vi "MCP23S17_Get.vi"(5 "RF":T1 items=["RF_0", "RF_1", "RF_2", "RF_3"], 6 "Addr":u32 format="%x", 7 "RFU":T2, 8 "Error_In":errorcluster, 10 "Auto_Sel_Rsrc?":bool=TRUE, 11 "VISA_Rsrc_In":refnum<visa-resource-name>) -> (0 "Error_Out":errorcluster, 2 "Data":u32 format="%x", 3 "VISA_Rsrc_Out":refnum<visa-resource-name>)   [LabVIEW 2018]
uses:
  Types/RFU.ctl
  Types/RF.ctl
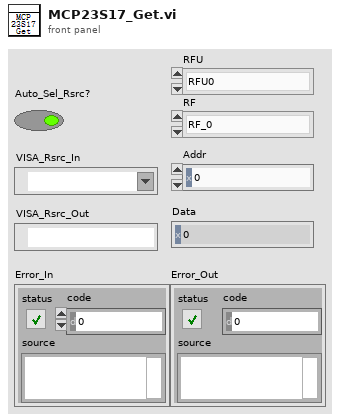
[diagram p1: front panel]
types:
  T1 = typedef "RF.ctl" = u16
  T2 = typedef "RFU.ctl" = enum8{"RFU0", "RFU1", "RFU2", "RFU3", "RFU4"}
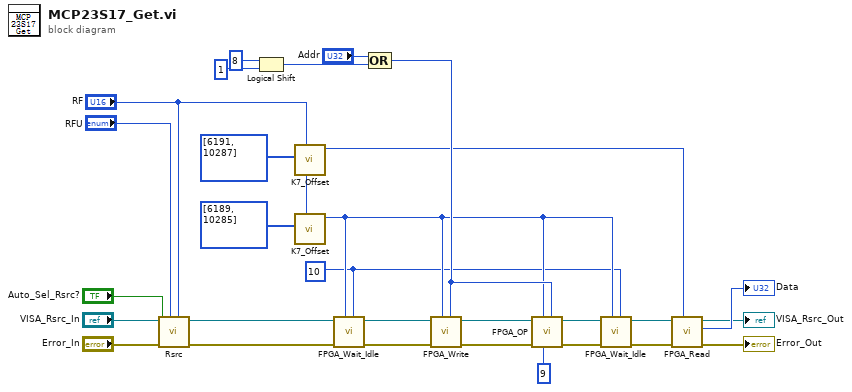
[diagram p0: block diagram]
diagram:
  w9 = u32 10 ("Bit_Offset")
  n1 = call "Rsrc.vi"("RF"="RF", "RFU"="RFU", "Error_In"="Error_In", "Auto_Sel_Rsrc?"="Auto_Sel_Rsrc?", "VISA_Rsrc_In"="VISA_Rsrc_In") -> ("Error_Out"=w28:errorcluster, "VISA_Rsrc_Out"=w24:refnum<visa-resource-name>)  [unwired: 5 in]
  n2 = Logical Shift(y=i16 8, x=u32 1 ("Bit_Offset")) -> (x << y=w19:u32)
  n3 = call "K7_Offset.vi"("RF"="RF", "Offset"=u32[] [6191, 10287]) -> ("Offset"=w5:u32)  [unwired: 9 in]
  n4 = call "K7_Offset.vi"("RF"="RF", "Offset"=u32[] [6189, 10285]) -> ("Offset"=w10:u32)  [unwired: 9 in]
  n5 = call "FPGA_Wait_Idle.vi"("Bit_Offset"=w9, "Offset"=w10, "Error_In"=w28, "VISA_Rsrc_In"=w24) -> ("Error_Out"=w17:errorcluster, "VISA_Rsrc_Out"=w18:refnum<visa-resource-name>)  [unwired: 6 in]
  n6 = Compound Arithmetic op=OR("Addr", w19) -> (w14:u32)
  n7 = call "FPGA_Write.vi"("Value"=w14, "Offset"=w10, "Error_In"=w17, "VISA_Rsrc_In"=w18) -> ("Error_Out"=w15:errorcluster, "VISA_Rsrc_Out"=w16:refnum<visa-resource-name>)  [unwired: 6 in]
  n8 = call "FPGA_OP.vi"("Origin_Value"=w14, "OP_Offset"=u32 9, "Offset"=w10, "Error_In"=w15, "VISA_Rsrc_In"=w16) -> ("Error_Out"=w11:errorcluster, "VISA_Rsrc_Out"=w12:refnum<visa-resource-name>)  [unwired: 5 in]
  n9 = call "FPGA_Wait_Idle.vi"("Bit_Offset"=w9, "Offset"=w10, "Error_In"=w11, "VISA_Rsrc_In"=w12) -> ("Error_Out"=w7:errorcluster, "VISA_Rsrc_Out"=w8:refnum<visa-resource-name>)  [unwired: 6 in]
  n10 = call "FPGA_Read.vi"("Offset"=w5, "Error_In"=w7, "VISA_Rsrc_In"=w8) -> ("Error_Out"=→"Error_Out":errorcluster, "Value"=→"Data":u32, "VISA_Rsrc_Out"=→"VISA_Rsrc_Out":refnum<visa-resource-name>)  [unwired: 6 in]
